vi "Sleep HL.vi"(8 "error in (no error)":errorcluster, 10 "event data":u8, 11 "event cluster":T1) -> (0 "error out":errorcluster)   [LabVIEW 2020, in "FCR100.lvlib"]
uses:
  FCR100.lvlib
  Device state -- enum.ctl
  Wake HL data -- cluster.ctl
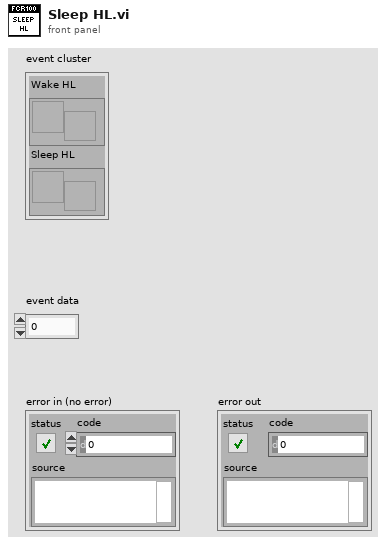
[diagram p1: front panel]
types:
  T1 = cluster{"Wake HL":refnum<user-event>, "Sleep HL":refnum<user-event>}
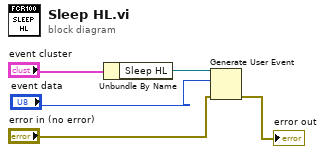
[diagram p0: block diagram]
diagram:
  n1 = Unbundle By Name("event cluster") -> ("Sleep HL"=w3:refnum<user-event>)
  n2 = Generate User Event(user event=w3, event data cluster="event data", error in="error in (no error)") -> (error out=→"error out":errorcluster)  [unwired: 1 in, 1 out]
